vi "CleanUp.vi"(0 "object in":refnum<class "Application.lvclass">, 5 "error in (no error)":errorcluster) -> (14 "object out":refnum<class "Application.lvclass">, 19 "error out":errorcluster)   [LabVIEW 2019, in "Application.lvclass"]
uses:
  Application.lvclass
  Application.lvclass/Application.ctl
  Hamamatsu_class/Hamamatsu.lvclass
  TDMSLogger_class/TDMSLogger.lvclass
  MTec_class/MTec.lvclass
  InstrumentBase_class/AD2_SDK_class/InstrumentBase.lvclass
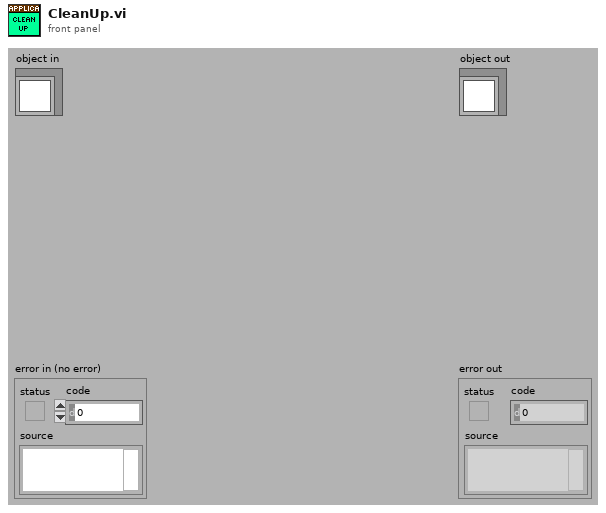
[diagram p1: front panel]
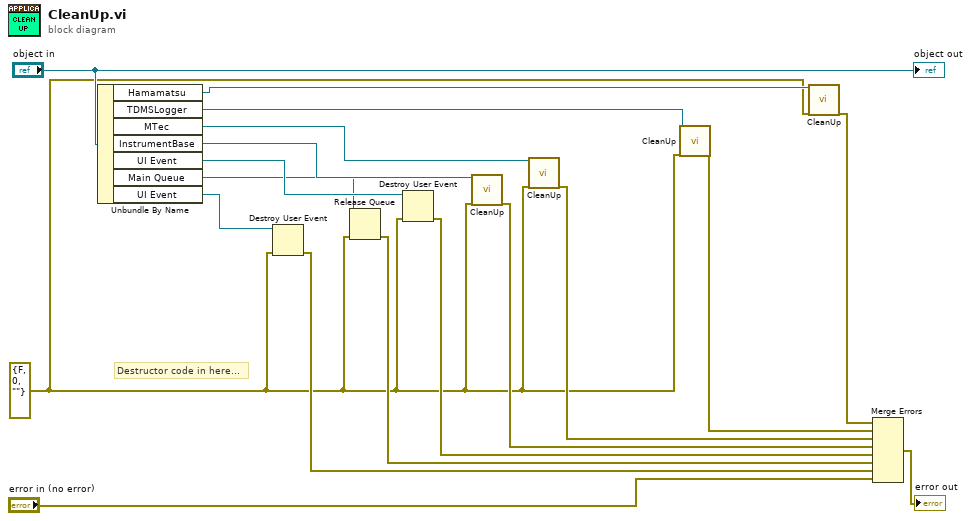
[diagram p0: block diagram]
diagram:
  w1 = errorcluster {"status"=FALSE, "code"=0, "source"=""} ("error in (no error)")
  # "Destructor code in here..."
  n1 = Unbundle By Name("object in") -> ("Hamamatsu"=w3:refnum<class "Hamamatsu.lvclass">, "TDMSLogger"=w5:refnum<class "TDMSLogger.lvclass">, "MTec"=w16:refnum<class "MTec.lvclass">, "InstrumentBase"=w15:refnum<class "InstrumentBase.lvclass">, "UI Event"=w14:refnum<user-event>, "Main Queue"=w13:refnum<queue>, "UI Event"=w12:refnum<user-event>)
  n2 = Destroy User Event(user event=w12, error in=w1) -> (error out=w7:errorcluster)
  n3 = Release Queue(queue=w13, error in (no error)=w1) -> (error out=w8:errorcluster)  [unwired: 1 in, 2 out]
  n4 = Destroy User Event(user event=w14, error in=w1) -> (error out=w9:errorcluster)
  n5 = call-dynamic "CleanUp.vi"("object in"=w15, "error in (no error)"=w1) -> ("error out"=w10:errorcluster)  [unwired: 16 in, 1 out]
  n6 = call-dynamic "CleanUp.vi"("object in"=w16, "error in (no error)"=w1) -> ("error out"=w11:errorcluster)  [unwired: 16 in, 1 out]
  n7 = call-dynamic "CleanUp.vi"("object in"=w5, "error in (no error)"=w1) -> ("error out"=w4:errorcluster)  [unwired: 16 in, 1 out]
  n8 = call-dynamic "CleanUp.vi"("object in"=w3, "error in (no error)"=w1) -> ("error out"=w2:errorcluster)  [unwired: 16 in, 1 out]
  n9 = Merge Errors(w2, w4, w11, w10, w9, w8, w7, "error in (no error)") -> (→"error out":errorcluster)
  "object out" <- "object in"
